vi "Extract Factors from INI Strings.vi"(1 "String":string) -> (0 "Conversion Factors":cluster{"Span":dbl, "Zero":dbl}[](array[cluster]) {"Zero" format="%.15f"; "Span" format="%.15f"})   [LabVIEW 2023]
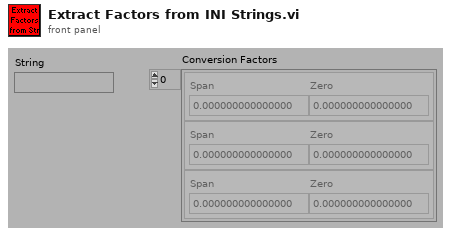
[diagram p1: front panel]
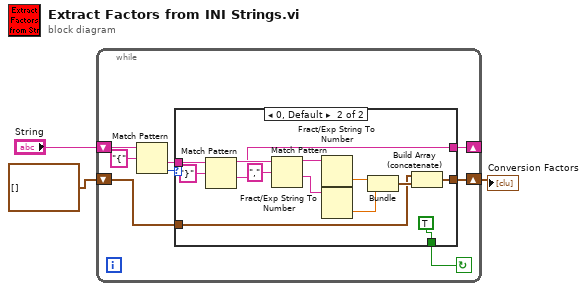
[diagram p0: block diagram]
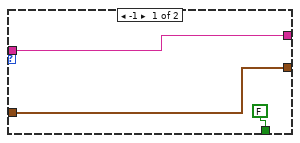
[diagram p2: hidden frame]
diagram:
  n1 = while {
    shift-right: [w8] -> _
    shift-left: "String" -> [w10]
    shift-right: [w7] -> w1
    shift-left: cluster{dbl, dbl}[] [] -> [w6]
    stop <- w4 continue-if-true
    n2 = Match Pattern(string=w10, regular expression="{") -> (after substring=w9:string, offset past match=w5:i32)  [unwired: 1 in, 2 out]
    n3 = case shown="0, Default" w5 {
      tunnel: w9 -> [w14 w27]
      tunnel: [w14 w19] -> w8
      tunnel: [w13 w17] -> w7
      tunnel: w6 -> [w13 w16]
      tunnel: [FALSE TRUE] -> w4
      frame -1 {
      }
      frame 0, Default {
        n4 = Match Pattern(string=w27, regular expression="}") -> (before substring=w25:string, after substring=w19:string)  [unwired: 1 in, 2 out]
        n5 = Match Pattern(string=w25, regular expression=",") -> (before substring=w23:string, after substring=w22:string)  [unwired: 1 in, 2 out]
        n6 = Fract/Exp String To Number(string=w23) -> (number=w21:dbl)  [unwired: 3 in, 1 out]
        n7 = Fract/Exp String To Number(string=w22) -> (number=w20:dbl)  [unwired: 3 in, 1 out]
        n8 = Bundle(w21, w20) -> (w18:cluster{dbl, dbl})  [unwired: 1 in]
        n9 = Build Array (concatenate)(w16, w18) -> (w17:cluster{dbl, dbl}[])
      }
    }
  }
  "Conversion Factors" <- w1
